vi "Write Channels.vi"(8 "error in":errorcluster, 10 "channels":refnum<class "Channel.lvclass">[](array[class]), 11 "module in":refnum<class "Module.lvclass">) -> (0 "error out":errorcluster, 3 "module out":refnum<class "Module.lvclass">)   [LabVIEW 2020, in "Scan Engine Scripting.lvlib" / "Module.lvclass"]
uses:
  Module.lvclass
  Channel Classes/Channel/Channel.lvclass
  Module.lvclass/Module.ctl
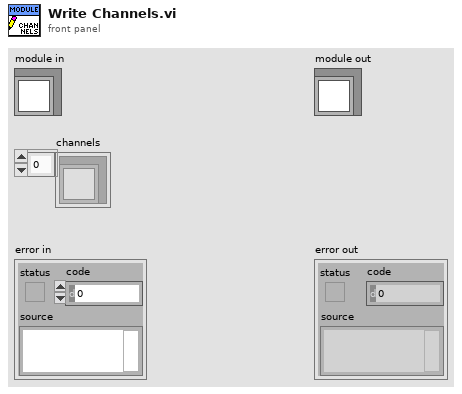
[diagram p1: front panel]
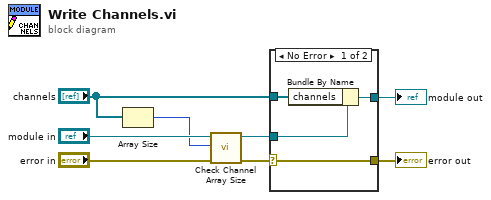
[diagram p0: block diagram]
diagram:
  n1 = Array Size(array="channels") -> (size(s)=w1:i32)
  n2 = call-dynamic "Check Channel Array Size.vi"("error in"="error in", "channel array size"=w1, "module in"="module in") -> ("error out"=w4:errorcluster, "module out"=w5:refnum<class "Module.lvclass">)  [unwired: 7 in]
  n3 = case shown="No Error" w4 {
    selector: w4 -> [w12 w13]
    tunnel: [w12 w13] -> w8
    tunnel: [w10 w14] -> w6
    tunnel: w5 -> [w11 w14]
    tunnel: "channels" -> [w9 _]
    frame No Error {
      n4 = Bundle By Name(cluster=w11, "channels"=w9) -> (w10:refnum<class "Module.lvclass">)
    }
    frame Error {
    }
  }
  "error out" <- w8
  "module out" <- w6
